vi "Resolve Actions.vi"(6 "Turn Results In":T1, 7 "Round":u32, 9 "Teams In":refnum<class "Team.lvclass">[](array[class]), 11 "Map in":refnum<class "Map.lvclass">) -> (1 "Teams":refnum<class "Team.lvclass">[](array[class]), 3 "Map out":refnum<class "Map.lvclass">, 4 "Turn Results":T1)   [LabVIEW 2020, in "SquareBattle.lvlib" / "Map.lvclass"]
uses:
  Map.lvclass
  Turn Results.ctl
  Team/Team.lvclass
  Map.lvclass/Map.ctl
  Position.ctl
  Square/Square.lvclass
  Direction Offsets Const.vi
  SquareBattle.lvlib
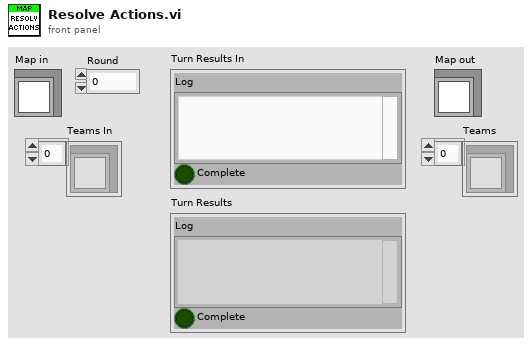
[diagram p1: front panel]
types:
  T1 = typedef "SquareBattle.lvlib/Turn Results.ctl" = cluster{"Log":string, "Complete":bool}
  T2 = typedef "SquareBattle.lvlib/Run Result.ctl" = cluster{"Action":T3, "Direction":T4, "Replication":refnum<class "Square.lvclass">}
  T3 = typedef "SquareBattle.lvlib/Action.ctl" = enum16{"Wait", "Move", "Attack", "Replicate"}
  T4 = typedef "SquareBattle.lvlib/Direction.ctl" = enum16{"NW", "N", "NE", "E", "SE", "S", "SW", "W"}
  T5 = typedef "SquareBattle.lvlib/Position.ctl" = cluster{"Row":i32, "Col":i32}
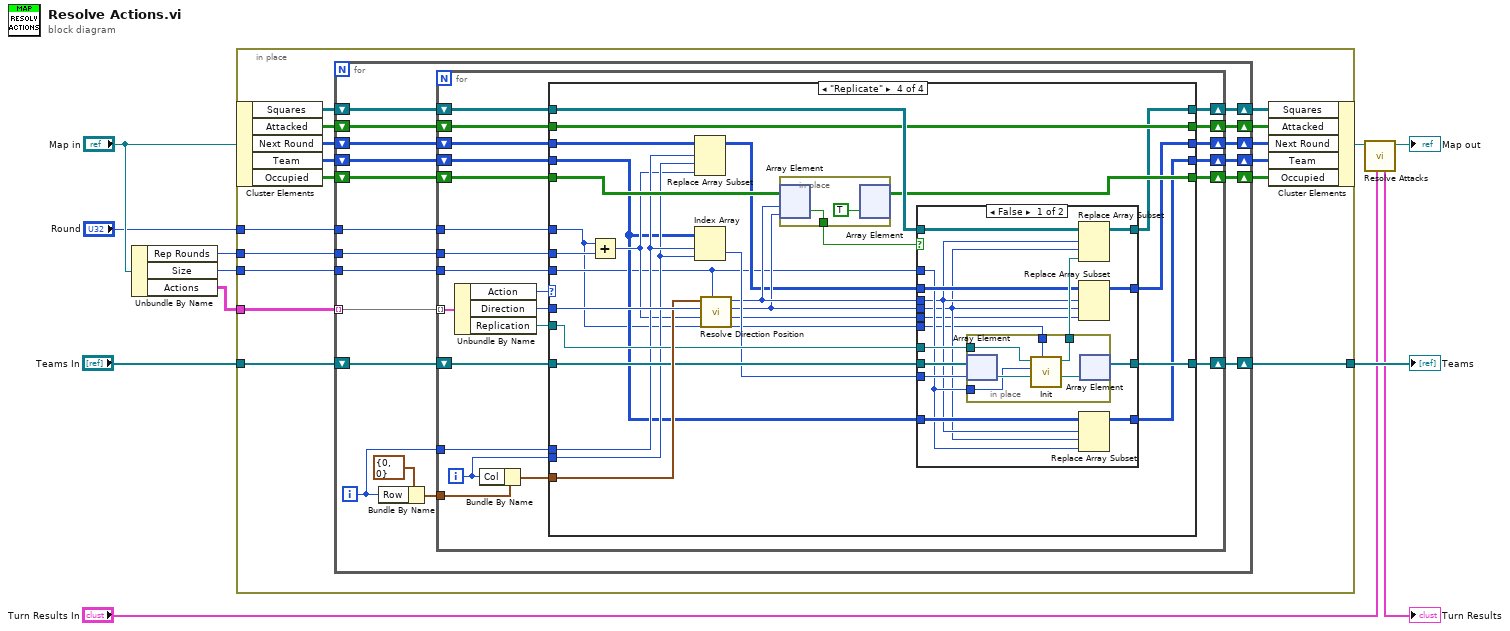
[diagram p0: block diagram]
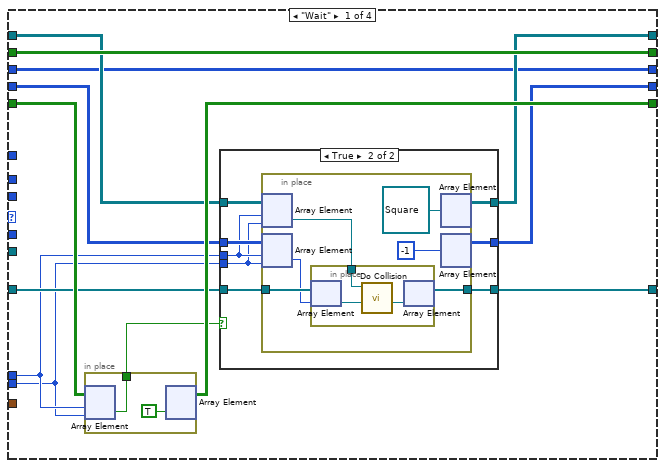
[diagram p2: hidden frame]
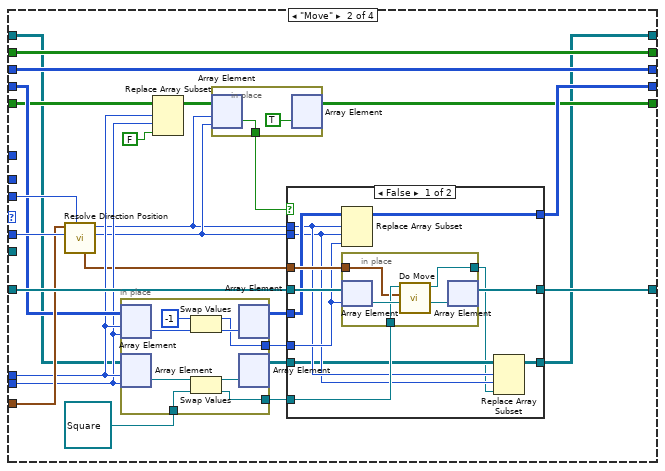
[diagram p4: hidden frame]
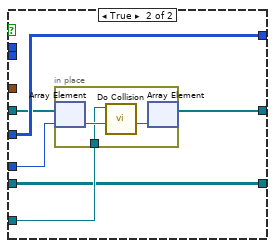
[diagram p5: hidden frame]
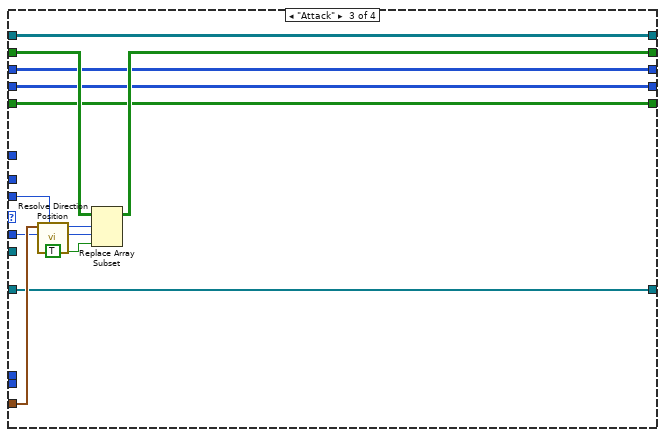
[diagram p6: hidden frame]
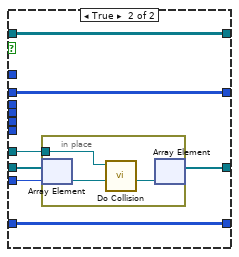
[diagram p7: hidden frame]
diagram:
  n1 = Unbundle By Name("Map in") -> ("Rep Rounds"=w6:u32, "Size"=w7:i32, "Actions"=w10:T2[][])
  n2 = in-place {
    in-place-border: w10 -> [w27]
    in-place-border: "Teams In" -> [w18]
    in-place-border: [w17] -> w8
    in-place-border: w7 -> [w14]
    in-place-border: w6 -> [w13]
    in-place-border: "Round" -> [w12]
    n3 = in-place-cluster #1("Map in") -> ("Squares"=w16:refnum<class "Square.lvclass">[][], "Attacked"=w26:bool[][], "Next Round"=w24:u32[][], "Team"=w23:i32[][], "Occupied"=w22:bool[][])
    n4 = for {
      shift-right: [w42] -> w25
      shift-left: w26 -> [w44]
      shift-right: [w43] -> w15
      shift-left: w16 -> [w45]
      tunnel: w27 -> [w46] mode=indexing
      shift-right: [w38] -> w19
      shift-left: w24 -> [w41]
      shift-right: [w37] -> w20
      shift-left: w23 -> [w40]
      shift-right: [w36] -> w21
      shift-left: w22 -> [w39]
      shift-right: [w34] -> w17
      shift-left: w18 -> [w35]
      tunnel: w14 -> [w30]
      tunnel: w13 -> [w29]
      tunnel: w12 -> [w28]
      i -> [w31]
      n5 = Bundle By Name(cluster=T5 {"Row"=0, "Col"=0} ("Position"), "Row"=w31) -> (w32:T5)
      n6 = for {
        shift-right: [w52] -> w42
        shift-left: w44 -> [w62]
        shift-right: [w51] -> w43
        shift-left: w45 -> [w61]
        tunnel: w46 -> [w69] mode=indexing
        shift-right: [w53] -> w38
        shift-left: w41 -> [w63]
        shift-right: [w50] -> w37
        shift-left: w40 -> [w64]
        shift-right: [w54] -> w36
        shift-left: w39 -> [w65]
        shift-right: [w59] -> w34
        shift-left: w35 -> [w60]
        tunnel: w32 -> [w57]
        tunnel: w31 -> [w58]
        tunnel: w30 -> [w49]
        tunnel: w29 -> [w48]
        tunnel: w28 -> [w47]
        i -> [w56]
        n7 = Unbundle By Name(w69) -> ("Action"=w68:T3, "Direction"=w67:T4, "Replication"=w66:refnum<class "Square.lvclass">)
        n8 = Bundle By Name(cluster=w57, "Col"=w56) -> (w55:T5)
        n9 = case shown="\"Replicate\"" w68 {
          tunnel: w67 -> [_ w130 w178 w204]
          tunnel: w66 -> [_ _ _ w201]
          tunnel: w65 -> [w82 w124 w168 w198]
          tunnel: w64 -> [w75 w125 w171 w183]
          tunnel: w63 -> [w72 w110 w172 w190]
          tunnel: w62 -> [w80 w109 w177 w192]
          tunnel: w61 -> [w78 w106 w173 w196]
          tunnel: w60 -> [w76 w127 w174 w202]
          tunnel: [w74 w113 w174 w191] -> w59
          tunnel: w58 -> [w71 w123 _ w189]
          tunnel: w56 -> [w70 w122 _ w188]
          tunnel: w55 -> [_ w126 w179 w203]
          tunnel: [w81 w108 w168 w193] -> w54
          tunnel: [w72 w110 w172 w185] -> w53
          tunnel: [w80 w109 w175 w192] -> w52
          tunnel: [w77 w107 w173 w187] -> w51
          tunnel: [w73 w111 w171 w182] -> w50
          tunnel: w49 -> [_ w129 w167 w181]
          tunnel: w48 -> [_ _ _ w200]
          tunnel: w47 -> [_ _ _ w180]
          frame "Wait" {
            n10 = in-place {
              in-place-border: [w104] -> w79
              n11 = in-place-array #2(w82, w71, w70) -> (w104:bool)
              n12 = in-place-array #2(TRUE ("element")) -> (w81:bool[][])  [unwired: 2 out]
            }
            n13 = case shown="True" w79 {
              tunnel: w78 -> [w83 w93]
              tunnel: w75 -> [w84 w92]
              tunnel: [w83 w91] -> w77
              tunnel: [w84 w90] -> w73
              tunnel: w76 -> [w85 w89]
              tunnel: [w85 w88] -> w74
              tunnel: w71 -> [_ w87]
              tunnel: w70 -> [_ w86]
              frame False {
              }
              frame True {
                n14 = in-place {
                  in-place-border: w89 -> [w98]
                  in-place-border: [w95] -> w88
                  n15 = in-place-array #3(w93, w87, w86) -> (w96:refnum<class "Square.lvclass">)
                  n16 = in-place-array #4(w92, w87, w86) -> (w97:i32)
                  n17 = in-place {
                    in-place-border: w96 -> [w100]
                    n18 = in-place-array #5(w98, w97) -> (w102:refnum<class "Team.lvclass">)
                    n19 = call "Do Collision.vi"("Team in"=w102, "Square"=w100) -> ("Team out"=w101:refnum<class "Team.lvclass">)  [unwired: 9 in]
                    n20 = in-place-array #5(w101) -> (w95:refnum<class "Team.lvclass">[])  [unwired: 1 out]
                  }
                  n21 = in-place-array #3(refnum<class "Square.lvclass"> refnum ("element")) -> (w91:refnum<class "Square.lvclass">[][])  [unwired: 2 out]
                  n22 = in-place-array #4(-1 ("element")) -> (w90:i32[][])  [unwired: 2 out]
                }
              }
            }
          }
          frame "Move" {
            n23 = call "Resolve Direction Position.vi"("Board Size"=w129, "Direction"=w130, "From"=w126) -> ("Col"=w115:i32, "Row"=w114:i32, "To"=w117:T5)  [unwired: 6 in]
            n24 = in-place {
              in-place-border: [w164] -> w128
              in-place-border: [w160] -> w119
              in-place-border: refnum<class "Square.lvclass"> refnum ("SquareBattle:Square") -> [w159]
              n25 = in-place-array #6(w125, w123, w122) -> (w163:i32)
              n26 = in-place-array #7(w106, w123, w122) -> (w166:refnum<class "Square.lvclass">)
              n27 = Swap Values(12:-1 ("element"), 14:w163) -> (1:w160:i32, 3:w162:i32)  [unwired: 1 in]
              n28 = Swap Values(12:w166, 14:w159) -> (1:w165:refnum<class "Square.lvclass">, 3:w164:refnum<class "Square.lvclass">)  [unwired: 1 in]
              n29 = in-place-array #6(w162) -> (w116:i32[][])  [unwired: 2 out]
              n30 = in-place-array #7(w165) -> (w112:refnum<class "Square.lvclass">[][])  [unwired: 2 out]
            }
            n31 = Replace Array Subset(array=w124, new element=FALSE ("new element/subarray"), index (row)=w123, index (col)=w122) -> (w121:bool[][])
            n32 = in-place {
              in-place-border: [w158] -> w118
              n33 = in-place-array #8(w121, w114, w115) -> (w158:bool)
              n34 = in-place-array #8(TRUE) -> (w108:bool[][])  [unwired: 2 out]
            }
            n35 = case shown="False" w118 {
              tunnel: w128 -> [w141 w151]
              tunnel: w127 -> [w142 w152]
              tunnel: w119 -> [w138 w148]
              tunnel: w117 -> [w140 _]
              tunnel: w116 -> [w139 w153]
              tunnel: w115 -> [w134 _]
              tunnel: w114 -> [w135 _]
              tunnel: [w137 w153] -> w111
              tunnel: [w136 w149] -> w113
              tunnel: w112 -> [w133 w150]
              tunnel: [w131 w150] -> w107
              frame False {
                n36 = Replace Array Subset(array=w139, new element=w138, index (row)=w135, index (col)=w134) -> (w137:i32[][])
                n37 = in-place {
                  in-place-border: w141 -> [w145]
                  in-place-border: w140 -> [w144]
                  in-place-border: [w143] -> w132
                  n38 = in-place-array #9(w142, w138) -> (w147:refnum<class "Team.lvclass">)
                  n39 = call "Do Move.vi"("Team in"=w147, "Position"=w144, "Square in"=w145) -> ("Team out"=w146:refnum<class "Team.lvclass">, "Square out"=w143:refnum<class "Square.lvclass">)  [unwired: 7 in]
                  n40 = in-place-array #9(w146) -> (w136:refnum<class "Team.lvclass">[])  [unwired: 1 out]
                }
                n41 = Replace Array Subset(array=w133, new element=w132, index (row)=w135, index (col)=w134) -> (w131:refnum<class "Square.lvclass">[][])
              }
              frame True {
                n42 = in-place {
                  in-place-border: w151 -> [w154]
                  n43 = in-place-array #10(w152, w148) -> (w156:refnum<class "Team.lvclass">)
                  n44 = call "Do Collision.vi"("Team in"=w156, "Square"=w154) -> ("Team out"=w155:refnum<class "Team.lvclass">)  [unwired: 9 in]
                  n45 = in-place-array #10(w155) -> (w149:refnum<class "Team.lvclass">[])  [unwired: 1 out]
                }
              }
            }
          }
          frame "Attack" {
            n46 = call "Resolve Direction Position.vi"("Board Size"=w167, "Direction"=w178, "From"=w179) -> ("Col"=w169:i32, "Row"=w170:i32)  [unwired: 6 in, 1 out]
            n47 = Replace Array Subset(array=w177, new element=TRUE ("new element/subarray"), index (row)=w170, index (col)=w169) -> (w175:bool[][])
          }
          frame "Replicate" {
            n48 = Add(x=w180, y=w200) -> (x+y=w184:u32)
            n49 = Replace Array Subset(array=w190, new element=w184, index (row)=w189, index (col)=w188) -> (w186:u32[][])
            n50 = Index Array(array=w183, index (row)=w189, index (col)=w188) -> (element=w199:i32)
            n51 = call "Resolve Direction Position.vi"("Board Size"=w181, "Direction"=w204, "From"=w203) -> ("Col"=w194:i32, "Row"=w195:i32)  [unwired: 6 in, 1 out]
            n52 = in-place {
              in-place-border: [w238] -> w197
              n53 = in-place-array #11(w198, w195, w194) -> (w238:bool)
              n54 = in-place-array #11(TRUE) -> (w193:bool[][])  [unwired: 2 out]
            }
            n55 = case shown="False" w197 {
              tunnel: w202 -> [w220 w232]
              tunnel: w201 -> [w219 w231]
              tunnel: w199 -> [w218 w230]
              tunnel: w181 -> [w210 _]
              tunnel: w196 -> [w217 w233]
              tunnel: w195 -> [w209 _]
              tunnel: w194 -> [w208 _]
              tunnel: [w215 w233] -> w187
              tunnel: [w214 w229] -> w191
              tunnel: w186 -> [w213 w228]
              tunnel: [w212 w228] -> w185
              tunnel: w184 -> [w207 _]
              tunnel: w183 -> [w211 w227]
              tunnel: [w206 w227] -> w182
              tunnel: w180 -> [w205 _]
              frame False {
                n56 = in-place {
                  in-place-border: w219 -> [w224]
                  in-place-border: w210 -> [w225]
                  in-place-border: [w222] -> w216
                  in-place-border: w205 -> [w221]
                  n57 = in-place-array #12(w220, w218) -> (w226:refnum<class "Team.lvclass">)
                  n58 = call "Init.vi"("Round"=w221, "Team in"=w226, "Board Size"=w225, "Square in"=w224) -> ("Team out"=w223:refnum<class "Team.lvclass">, "Square out"=w222:refnum<class "Square.lvclass">)  [unwired: 6 in]
                  n59 = in-place-array #12(w223) -> (w214:refnum<class "Team.lvclass">[])  [unwired: 1 out]
                }
                n60 = Replace Array Subset(array=w217, new element=w216, index (row)=w209, index (col)=w208) -> (w215:refnum<class "Square.lvclass">[][])
                n61 = Replace Array Subset(array=w213, new element=w207, index (row)=w209, index (col)=w208) -> (w212:u32[][])
                n62 = Replace Array Subset(array=w211, new element=w210, index (row)=w209, index (col)=w208) -> (w206:i32[][])
              }
              frame True {
                n63 = in-place {
                  in-place-border: w231 -> [w235]
                  n64 = in-place-array #13(w232, w230) -> (w236:refnum<class "Team.lvclass">)
                  n65 = call "Do Collision.vi"("Team in"=w236, "Square"=w235) -> ("Team out"=w234:refnum<class "Team.lvclass">)  [unwired: 9 in]
                  n66 = in-place-array #13(w234) -> (w229:refnum<class "Team.lvclass">[])  [unwired: 1 out]
                }
              }
            }
          }
        }
      }
    }
    n67 = in-place-cluster #1("Squares"=w15, "Attacked"=w25, "Next Round"=w19, "Team"=w20, "Occupied"=w21) -> (w4:refnum<class "Map.lvclass">)
  }
  "Teams" <- w8
  n68 = call "Resolve Attacks.vi"("Turn Results In"="Turn Results In", "Map in"=w4) -> ("Map out"=→"Map out":refnum<class "Map.lvclass">, "Turn Results"=→"Turn Results":T1)  [unwired: 8 in]
